vi "Update Scroll Length.vi"(8 "error in (no error)":errorcluster, 11 "PanelArray in":refnum<class "PanelArray.lvclass">) -> (0 "error out":errorcluster, 3 "PanelArray out":refnum<class "PanelArray.lvclass">)   [LabVIEW 2018, in "OOPanel.lvlib" / "PanelArray.lvclass"]
uses:
  PanelArray.lvclass
  PanelArray.lvclass/PanelArray.ctl
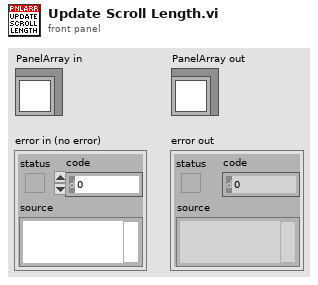
[diagram p1: front panel]
types:
  T1 = typedef "OOPanel.lvlib/PanelArray.lvclass/Ref Data.ctl" = cluster{"State":T2, "Refs":T3, "Events":T4, "Scrolling":T5, "Panels":T6}
  T2 = typedef "OOPanel.lvlib/PanelArray.lvclass/State.ctl" = cluster{"Defer Updates":bool, "Running":bool, "Dynamic Sizing":bool, "Borders":bool}
  T3 = typedef "OOPanel.lvlib/PanelArray.lvclass/Refs.ctl" = cluster{"SubPanels":refnum<vi>[], "Scrollbar":refnum<vi>, "Owning Panel":refnum<vi>}
  T4 = typedef "OOPanel.lvlib/PanelArray.lvclass/Events.ctl" = cluster{"Close":refnum<user-event>}
  T5 = typedef "OOPanel.lvlib/PanelArray.lvclass/Scrolling.ctl" = cluster{"Size":i32, "Max":i32, "Current":i32, "Top Index":i32, "Heights":i32[]}
  T6 = typedef "OOPanel.lvlib/PanelArray.lvclass/Panels.ctl" = cluster{"All":refnum<class "Panel.lvclass">[], "Visible":refnum<class "Panel.lvclass">[], "Blank":refnum<class "ArrayBlank.lvclass">}
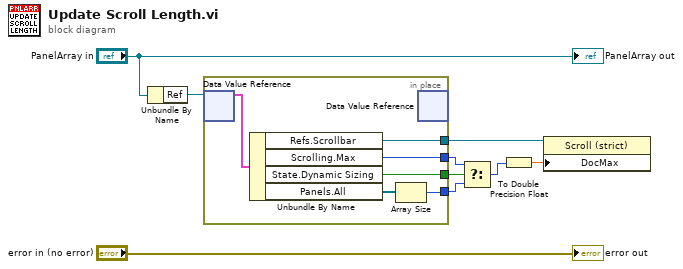
[diagram p0: block diagram]
diagram:
  n1 = Unbundle By Name("PanelArray in") -> ("Ref"=w8:refnum<data-value>)
  n2 = in-place {
    in-place-border: [w14] -> w6
    in-place-border: [w13] -> w3
    in-place-border: [w11] -> w2
    in-place-border: [w10] -> w4
    n3 = in-place-dvr #1(w8) -> (w15:T1)  [unwired: 1 out]
    n4 = Unbundle By Name(w15) -> ("Refs.Scrollbar"=w14:refnum<vi>, "Scrolling.Max"=w13:i32, "State.Dynamic Sizing"=w10:bool, "Panels.All"=w12:refnum<class "Panel.lvclass">[])
    n5 = Array Size(array=w12) -> (size(s)=w11:i32)
    n6 = in-place-dvr #1() -> ()  [unwired: 1 in, 2 out]
  }
  n7 = Select(t=w3, s=w4, f=w2) -> (s? t:f=w1:i32)
  n8 = To Double Precision Float(number=w1) -> (double precision float=w5:dbl)
  n9 = property class="Scroll (strict)"(reference=w6, "DocMax"=w5) -> ()  [unwired: 1 in, 2 out]
  "error out" <- "error in (no error)"
  "PanelArray out" <- "PanelArray in"
